vi "quicktest_withoutIPR.vi"() -> ()   [LabVIEW 2009]
panel:
  out "LS_Hd":u32
  out "number 2":u32
  in  "VC_EN":bool=TRUE
  in  "VC_3NS":bool
  in  "VC_2NS":bool
  in  "VC_L":bool
  in  "VC_H":bool
  in  "VC 0.25ns":bool
  in  "Boolean 2":bool=TRUE
  out "number":u32
  out "LS_L":string
  out "LS_H":string
  in  "LS_H":i32=72
  in  "reg":i32
  out "data out 2":string
  out "data out":string
  out "x/y":dbl
  in  "n":i32=255
  in  "Boolean":bool=TRUE
  in  "x":i32=4095
  out "error out":errorcluster
  in  "Address":i32
  out "DAC0 Value":i32
  in  "stop":bool
  out "IPR value":i32
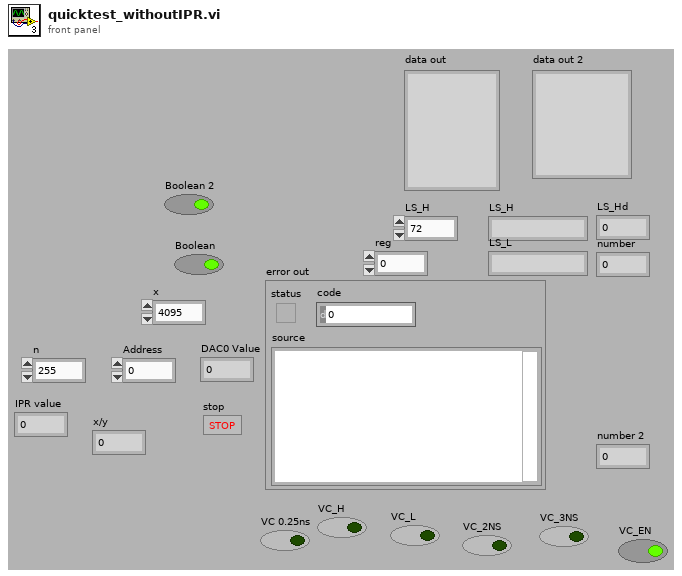
[diagram p1: front panel]
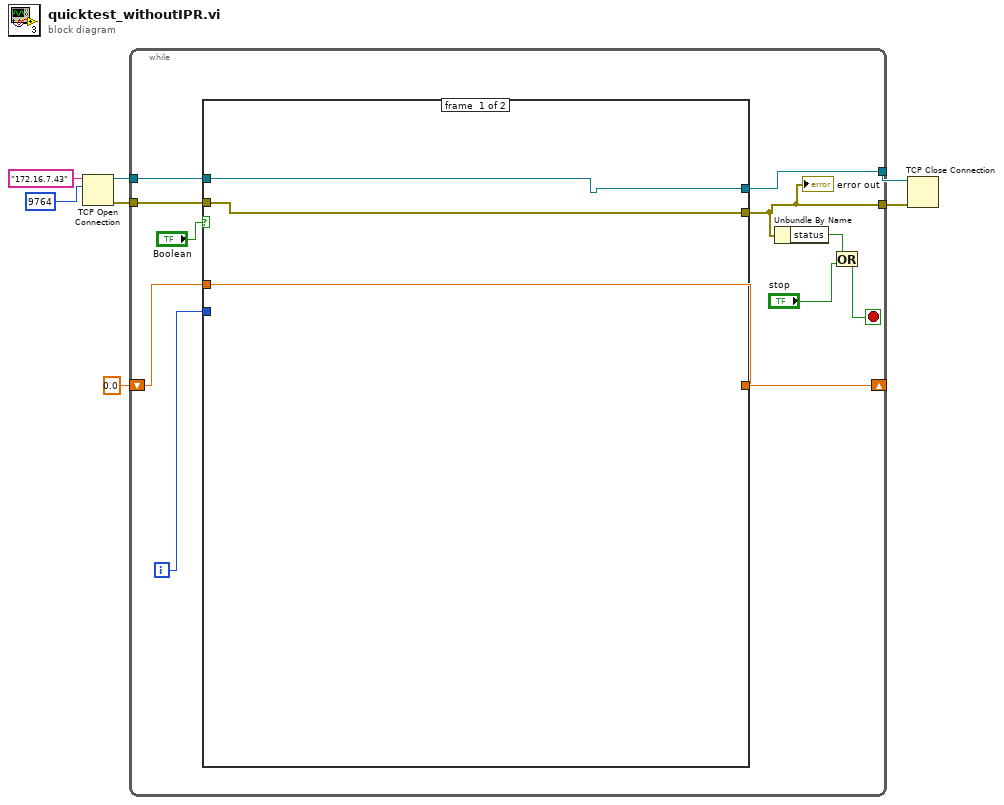
[diagram p0: block diagram]
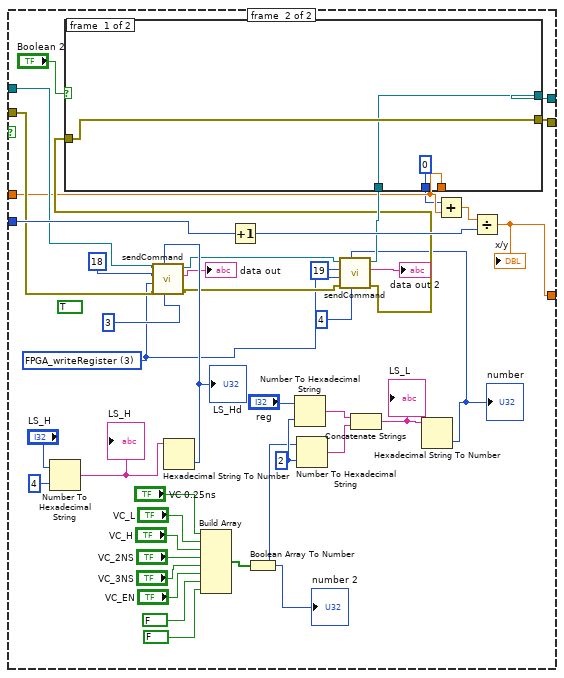
[diagram p2: hidden frame]
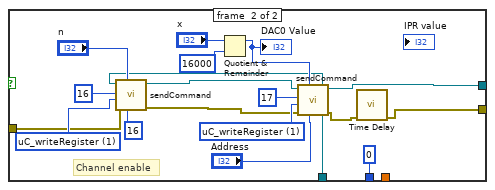
[diagram p3: hidden frame]
diagram:
  n1 = TCP Open Connection(address="172.16.7.43", remote port or service name=u16 9764) -> (connection ID=w7:refnum<k5>, error out=w4:errorcluster)  [unwired: 3 in]
  n2 = while {
    tunnel: w7 -> [w17]
    tunnel: w4 -> [w18]
    tunnel: [w14] -> w3
    tunnel: [w15] -> w2
    shift-right: [w10] -> _
    shift-left: 0.0 -> [w9]
    i -> [w8]
    stop <- w13 stop-if-true
    n3 = case shown="True" "Boolean" {
      tunnel: [w20 w53] -> w14
      tunnel: w18 -> [w20 w51]
      tunnel: w17 -> [w21 w50]
      tunnel: [w21 w52] -> w15
      tunnel: [w19 w33] -> w10
      tunnel: w9 -> [w19 w36]
      tunnel: w8 -> [_ w63]
      frame #0 {
      }
      frame #1 {
        w54 = i16 2 ("width (-)")
        (unwired) TRUE ("Send")
        w41 = u16 3 items=["sendCommand"=9, "FPGA_writeRegister"=3, "FPGA_readRegister"=2, "uC_writeRegister"=1, "uC_readRegister"=0] ("Action")
        n4 = Number To Hexadecimal String(1:i16 4 ("width (-)"), 2:"LS_H") -> (0:w58:string)
        "LS_H" <- w58
        n5 = Hexadecimal String To Number(string=w58) -> (number=w48:u32)  [unwired: 2 in, 1 out]
        "LS_Hd" <- w48
        n6 = call "sendCommand.vi"("Address"=3, "Data"=w48, "error in"=w51, "Action"=w41, "id_in"=18 ("id"), "connection ID"=w50) -> ("error out"=w43:errorcluster, "Data out"=→"data out":string, "connection ID out"=w39:refnum<k5>)  [unwired: 1 in, 2 out]
        n7 = Build Array("VC 0.25ns", "VC_L", "VC_H", "VC_2NS", "VC_3NS", "VC_EN", FALSE ("element"), FALSE ("element")) -> (w23:bool[])
        n8 = Increment(x=w63) -> (x+1=w62:i32)
        n9 = Boolean Array To Number(Boolean array=w23) -> (number=w22:u32)
        "number 2" <- w22
        n10 = Number To Hexadecimal String(1:w54, 2:"reg") -> (0:w56:string)
        n11 = Number To Hexadecimal String(1:w54, 2:w22) -> (0:w57:string)
        n12 = Concatenate Strings(w56, w57) -> (w61:string)
        "LS_L" <- w61
        n13 = Hexadecimal String To Number(string=w61) -> (number=w38:u32)  [unwired: 2 in, 1 out]
        "number" <- w38
        n14 = call "sendCommand.vi"("Address"=4, "Data"=w38, "error in"=w43, "Action"=w41, "id_in"=19 ("id"), "connection ID"=w39) -> ("error out"=w44:errorcluster, "Data out"=→"data out 2":string, "connection ID out"=w45:refnum<k5>)  [unwired: 1 in, 2 out]
        n15 = case shown="True" "Boolean 2" {
          tunnel: w36 -> [_ _]
          tunnel: [w66 w69] -> w53
          tunnel: [w65 w68] -> w52
          tunnel: w45 -> [w65 w71]
          tunnel: w44 -> [w66 w70]
          tunnel: [0 ("IPR value") 0 ("IPR value")] -> w35
          frame #0 {
          }
          frame #1 {
            w80 = u16 1 items=["sendCommand"=9, "FPGA_writeRegister"=3, "FPGA_readRegister"=2, "uC_writeRegister"=1, "uC_readRegister"=0] ("Action")
            w83 = u16 1 items=["sendCommand"=9, "FPGA_writeRegister"=3, "FPGA_readRegister"=2, "uC_writeRegister"=1, "uC_readRegister"=0] ("Action")
            # "Channel enable"
            n16 = call "sendCommand.vi"("Address"=16, "Data"="n", "error in"=w70, "Action"=w80, "id_in"=16 ("id"), "connection ID"=w71) -> ("error out"=w78:errorcluster, "connection ID out"=w79:refnum<k5>)  [unwired: 1 in, 3 out]
            n17 = Quotient & Remainder(x="x", y=16000) -> (x-y*floor(x/y)=w77:i32)  [unwired: 1 out]
            "DAC0 Value" <- w77
            n18 = call "sendCommand.vi"("Address"="Address", "Data"=w77, "error in"=w78, "Action"=w83, "id_in"=17 ("id"), "connection ID"=w79) -> ("error out"=w74:errorcluster, "connection ID out"=w68:refnum<k5>)  [unwired: 1 in, 3 out]
            n19 = call "Time Delay"("error in (no error)"=w74) -> ("error out"=w69:errorcluster)  [unwired: 10 in]
          }
        }
        n20 = Add(x=w35, y=w36) -> (x+y=w34:dbl)
        n21 = Divide(x=w34, y=w62) -> (x/y=w33:dbl)
        "x/y" <- w33
      }
    }
    "error out" <- w14
    n22 = Unbundle By Name(w14) -> ("status"=w12:bool)
    n23 = Or(x=w12, y="stop") -> (x .or. y?=w13:bool)
  }
  n24 = TCP Close Connection(connection ID=w2, error in (no error)=w3) -> ()  [unwired: 1 in, 2 out]
